vi "CMN_CallGeometry.vi"(0 "Command":string, 11 "error in (no error)":errorcluster) -> (4 "ImmedReplyString":string, 15 "error out":errorcluster)   [LabVIEW 2016]
panel:
  in  "VI path":path=path "/home/ArcVIEW/Modules/GEOM/public/vis"
  in  "AVAPP Cmd Proc":refnum<vi>
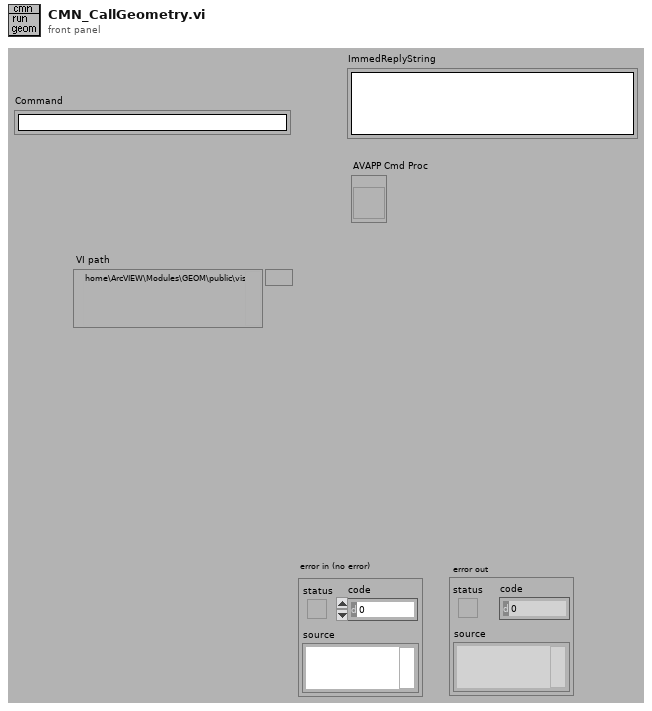
[diagram p1: front panel]
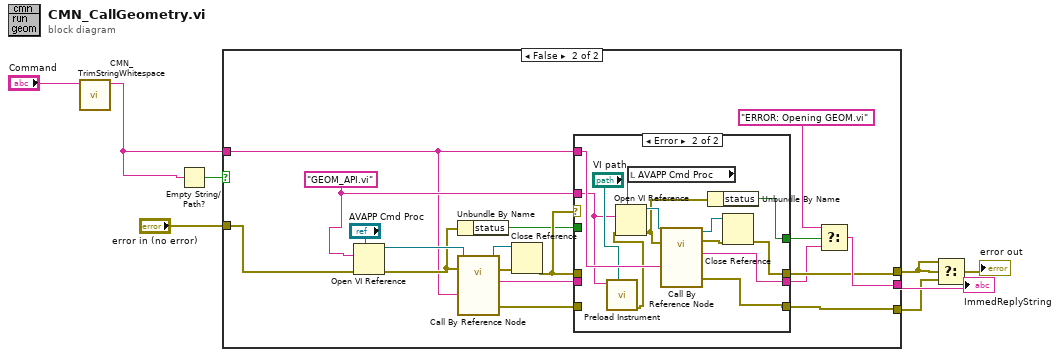
[diagram p0: block diagram]
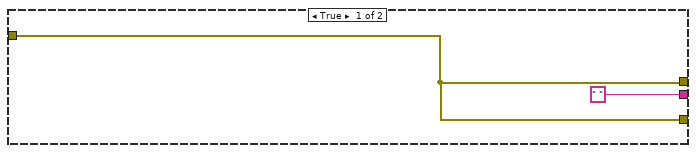
[diagram p2: hidden frame]
diagram:
  n1 = call "CMN_TrimStringWhitespace.vi"("string"="Command") -> ("trimmed string"=w4:string)  [unwired: 1 in, 8 out]
  n2 = Empty String/Path?(string/path=w4) -> (empty?=w5:bool)
  n3 = case shown="False" w5 {
    tunnel: [" " w22] -> w8
    tunnel: [w9 w19] -> w3
    tunnel: "error in (no error)" -> [w9 w26]
    tunnel: w4 -> [_ w11]
    tunnel: [w9 w17] -> w2
    frame True {
    }
    frame False {
      w13 = "GEOM_API.vi"
      n4 = Open VI Reference(type specifier VI Refnum (for type only)="AVAPP Cmd Proc", vi path=w13, error in (no error)=w26) -> (vi reference=w28:refnum<vi>, error out=w23:errorcluster)  [unwired: 3 out]
      n5 = Unbundle By Name(w23) -> ("status"=w16:bool)
      n6 = call-by-ref "Call By Reference Node"(reference=w28, error in=w23, "Cmd"=w11) -> (reference out=w24:refnum<vi>, error out=w25:errorcluster, "ImmedReplyString"=w15:string, 15:"error out"=w18:errorcluster)  [unwired: 13 in]
      n7 = Close Reference(reference=w24, error in (no error)=w25) -> (error out=w20:errorcluster)
      n8 = case shown="Error" w20 {
        tunnel: w20 -> [w32 _]
        tunnel: [w32 w41] -> w19
        tunnel: w18 -> [w31 _]
        tunnel: [w31 w37] -> w17
        tunnel: w16 -> [w29 _]
        tunnel: w15 -> [w30 _]
        tunnel: [w30 w40] -> w14
        tunnel: w13 -> [_ w33]
        tunnel: [w29 w38] -> w12
        tunnel: w11 -> [_ w36]
        frame No Error {
        }
        frame Error {
          n9 = call <vilib>:"Preload Instrument.vi"("VI path"="VI path", "VI name"=w33) -> ("error out"=w34:errorcluster)  [unwired: 1 in, 8 out]
          n10 = local read "AVAPP Cmd Proc"() -> (w45:refnum<vi>)
          n11 = Open VI Reference(type specifier VI Refnum (for type only)=w45, vi path=w33, error in (no error)=w34) -> (vi reference=w44:refnum<vi>, error out=w39:errorcluster)  [unwired: 3 out]
          n12 = call-by-ref "Call By Reference Node"(reference=w44, error in=w39, "Cmd"=w36) -> (reference out=w42:refnum<vi>, error out=w43:errorcluster, "ImmedReplyString"=w40:string, 15:"error out"=w37:errorcluster)  [unwired: 13 in]
          n13 = Unbundle By Name(w39) -> ("status"=w38:bool)
          n14 = Close Reference(reference=w42, error in (no error)=w43) -> (error out=w41:errorcluster)
        }
      }
      n15 = Select(t="ERROR: Opening GEOM.vi", s=w12, f=w14) -> (s? t:f=w22:string)
    }
  }
  "ImmedReplyString" <- w8
  n16 = Select(t=w3, s=w3, f=w2) -> (s? t:f=→"error out":errorcluster)
